vi "FGV_PSP - IPS120 Targets.vi"(4 "error in":errorcluster, 6 "Function":enum16{"write", "read"}(ring), 7 "Targets":T1) -> (0 "error out":errorcluster, 3 "Targets":T1)   [LabVIEW 2016, in "IPS-120.lvlib" / "IPS-120-API.lvlib"]
uses:
  IPS-120-API.lvlib
panel:
  # "Disabled calls to PSP 4/13/2018"
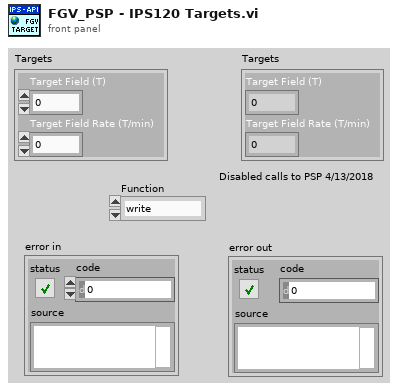
[diagram p1: front panel]
types:
  T1 = cluster{"Target Field (T)":dbl, "Target Field Rate (T/min)":dbl}
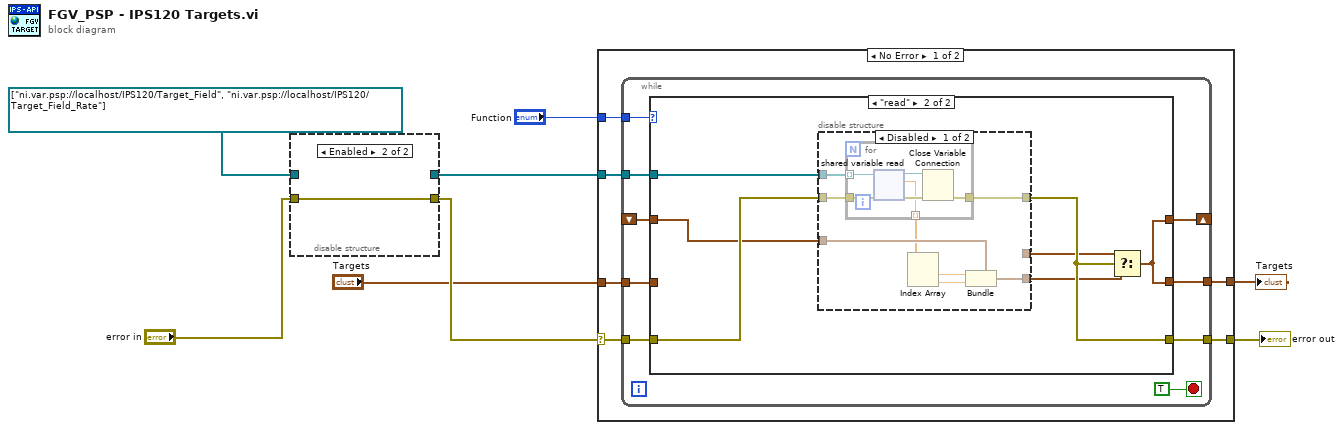
[diagram p0: block diagram]
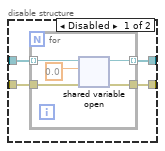
[diagram p2: hidden frame]
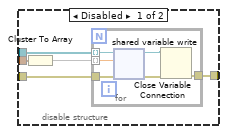
[diagram p4: hidden frame]
diagram:
  n1 = disable-structure shown="Enabled" {
    disable-tunnel: [w12 _] -> w6
    disable-tunnel: [w11 w18] -> w5
    disable-tunnel: "error in" -> [w10 w18]
    disable-tunnel: refnum<k21>[] ["ni.var.psp://localhost/IPS120/Target_Field", "ni.var.psp://localhost/IPS120/Target_Field_Rate"] -> [w9 _]
    frame Disabled {
      n2 = for {
        tunnel: [w17] -> w12 mode=indexing
        tunnel: [w16] -> w11
        tunnel: w10 -> [w15]
        tunnel: w9 -> [w14] mode=indexing
        n3 = shared-variable-open(w14, w15, 0.0) -> (w17:refnum<k21>, w16:errorcluster)  [unwired: 1 in]
      }
    }
    frame Enabled {
    }
  }
  n4 = case shown="No Error" w5 {
    selector: w5 -> [w24 w74]
    tunnel: [w23 w74] -> w8
    tunnel: [w22 w73] -> w2
    tunnel: "Function" -> [w21 _]
    tunnel: w6 -> [w20 _]
    tunnel: "Targets" -> [w19 w73]
    frame No Error {
      n5 = while {
        shift-right: [w28] -> _
        shift-left: _ -> [w27]
        tunnel: w24 -> [w32]
        tunnel: [w31] -> w23
        tunnel: [w30] -> w22
        tunnel: w21 -> [w29]
        tunnel: w20 -> [w26]
        tunnel: w19 -> [w25]
        stop <- TRUE stop-if-true
        n6 = case shown="\"read\"" w29 {
          tunnel: w32 -> [w36 w54]
          tunnel: [w37 w53] -> w31
          tunnel: [w34 w56] -> w30
          tunnel: [w34 w56] -> w28
          tunnel: w27 -> [_ w52]
          tunnel: w26 -> [w35 w55]
          tunnel: w25 -> [w34 _]
          frame "write", Default {
            n7 = disable-structure shown="Enabled" {
              disable-tunnel: [w42 w49] -> w37
              disable-tunnel: w36 -> [w41 w49]
              disable-tunnel: w35 -> [w40 _]
              disable-tunnel: w34 -> [w38 _]
              frame Disabled {
                n8 = Cluster To Array(cluster=w38) -> (array=w39:dbl[])
                n9 = for {
                  tunnel: [w47] -> w42
                  tunnel: w41 -> [w45]
                  tunnel: w40 -> [w44] mode=indexing
                  tunnel: w39 -> [w43] mode=indexing
                  n10 = shared-variable-write(w44, w45, w43) -> (w46:refnum<k21>, w48:errorcluster)
                  n11 = Close Variable Connection(8:w48, 11:w46) -> (0:w47:errorcluster)
                }
              }
              frame Enabled {
              }
            }
          }
          frame "read" {
            n12 = disable-structure shown="Disabled" {
              disable-tunnel: w55 -> [w64 _]
              disable-tunnel: w54 -> [w63 w71]
              disable-tunnel: [w62 w71] -> w53
              disable-tunnel: w52 -> [w61 w72]
              disable-tunnel: [w60 w72] -> w51
              disable-tunnel: [_ w72] -> w50
              frame Disabled {
                n13 = for {
                  tunnel: [w68] -> w62
                  tunnel: w64 -> [w67] mode=indexing
                  tunnel: w63 -> [w66]
                  tunnel: [w65] -> w59 mode=indexing
                  n14 = shared-variable-read(w67, w66) -> (w70:refnum<k21>, w69:errorcluster, w65:dbl)  [unwired: 1 out]
                  n15 = Close Variable Connection(8:w69, 11:w70) -> (0:w68:errorcluster)
                }
                n16 = Index Array(array=w59) -> (element #1=w58:dbl, element #2=w57:dbl)  [unwired: 2 in]
                n17 = Bundle(cluster=w61, "Target Field (T)"=w58, "Target Field Rate (T/min)"=w57) -> (w60:T1)
              }
              frame Enabled {
              }
            }
            n18 = Select(t=w50, s=w53, f=w51) -> (s? t:f=w56:T1)
          }
        }
      }
    }
    frame Error {
    }
  }
  "error out" <- w8
  "Targets" <- w2
